vi "util_prepare_XY_graph.vi"(4 "Y":dbl format="%#_13g", 6 "X":dbl format="%#_13g", 8 "Y array":dbl[](array[numeric]), 9 "X array":dbl[](array[numeric]), 10 "IsFirst":bool, 11 "XY Graph in":cluster{i32[], dbl[]}[](array[cluster])) -> (0 "Y array out":dbl[](array[numeric]), 1 "X array out":dbl[](array[numeric]), 3 "XY Graph out":cluster{"Array":dbl[], "Array":dbl[]}[](array[cluster]))   [LabVIEW 2016]
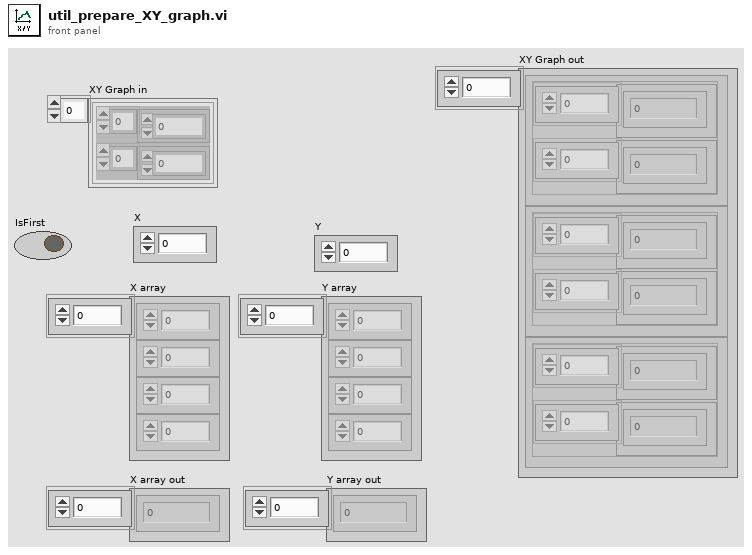
[diagram p1: front panel]
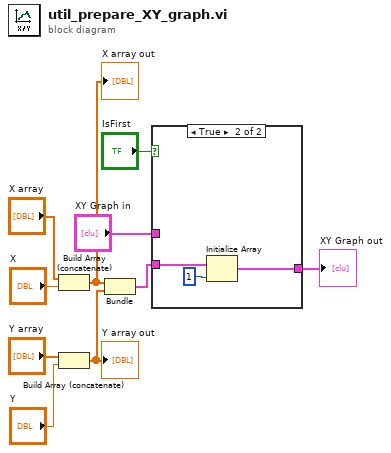
[diagram p0: block diagram]
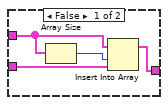
[diagram p2: hidden frame]
diagram:
  n1 = Build Array (concatenate)("X array", "X") -> (w10:dbl[])
  "X array out" <- w10
  n2 = Build Array (concatenate)("Y array", "Y") -> (w9:dbl[])
  "Y array out" <- w9
  n3 = Bundle(w10, w9) -> (w8:cluster{dbl[], dbl[]})  [unwired: 1 out]
  n4 = case shown="True" "IsFirst" {
    tunnel: "XY Graph in" -> [w13 _]
    tunnel: [w12 w15] -> w2
    tunnel: w8 -> [w11 w16]
    frame False {
      n5 = Array Size(array=w13) -> (size(s)=w14:i32)
      n6 = Insert Into Array(array=w13, index=w14, new element=w11) -> (w12:cluster{i32[], dbl[]}[])
    }
    frame True {
      n7 = Initialize Array(w16, 1 ("dimension size")) -> (w15:cluster{dbl[], dbl[]}[])
    }
  }
  "XY Graph out" <- w2
